vi "Get Last PString.vi"(0 "String":string) -> (1 "Last PString":string, 2 "PString Offset":i32)   [LabVIEW 2017, in "_reuse_openG.lvlib"]
doc: "Returns the last PString from the end of the string and the offset of the beginning of the string."
uses:
  _reuse_openG.lvlib
panel:
  # "[OpenG VI Tags] ***Do Not Remove***"
  # "Get Last PString.vi\n\nReturns the last PString from the end of the string and the offset of the beginn\n\nPlease visit http://www.OpenG.org to learn about the\nOpen Source LabVIEW software movement.\n\nNOTICE -- YOU MUST LEAVE THIS NOTICE IN PLACE.  PER THE TERMS OF THE LICENSE BELOW, YOU MAY SUBLICENSE THIS SOFTWARE \nIN ANY WAY THAT DOES NOT CONFLICT WITH THIS LICENSE.\n\n### BSD License (http://www.opensource.org/licenses/bsd-license.php) Begin ###\n \nCopyright (c) 2002, Jean-Pierre Drolet <drolet_jp@hotmail.com>\nCopyright (c) 2002-2006, Jim Kring <jim@jimkring.com>\n\nAll rights reserved.\n\nRedistribution and use in source and binary forms, with or without modification, are permitted provided that the following conditions are met:\n\n    * Redistributions of source code must retain the above copyright notice, this list of conditions and the following disclaimer.\n    * Redistributions in binary form must reproduce the above copyright notice, this list of conditions and the following disclaimer in the \n       documentation and/or other materials provided with the distribution.\n    * Neither the name of SciWare, James Kring, Inc., nor the names of its contributors may be used to endorse or promote products derived \n       from this software without specific prior written permission.\n\nTHIS SOFTWARE IS PROVIDED BY THE COPYRIGHT HOLDERS AND CONTRIBUTORS \"AS IS\" AND ANY EXPRESS OR IMPLIED WARRANTIES, \nINCLUDING, BUT NOT LIMITED TO, THE IMPLIED WARRANTIES OF MERCHANTABILITY AND FITNESS FOR A PARTICULAR PURPOSE ARE \nDISCLAIMED. IN NO EVENT SHALL THE COPYRIGHT OWNER OR CONTRIBUTORS BE LIABLE FOR ANY DIRECT, INDIRECT, INCIDENTAL,\n SPECIAL, EXEMPLARY, OR CONSEQUENTIAL DAMAGES (INCLUDING, BUT NOT LIMITED TO, PROCUREMENT OF SUBSTITUTE GOODS OR \nSERVICES; LOSS OF USE, DATA, OR PROFITS; OR BUSINESS INTERRUPTION) HOWEVER CAUSED AND ON ANY THEORY OF LIABILITY, \nWHETHER IN CONTRACT, STRICT LIABILITY, OR TORT (INCLUDING NEGLIGENCE OR OTHERWISE) ARISING IN ANY WAY OUT OF THE USE \nOF THIS SOFTWARE, EVEN IF ADVISED OF THE POSSIBILITY OF SUCH DAMAGE.\n\n### BSD License End ###"
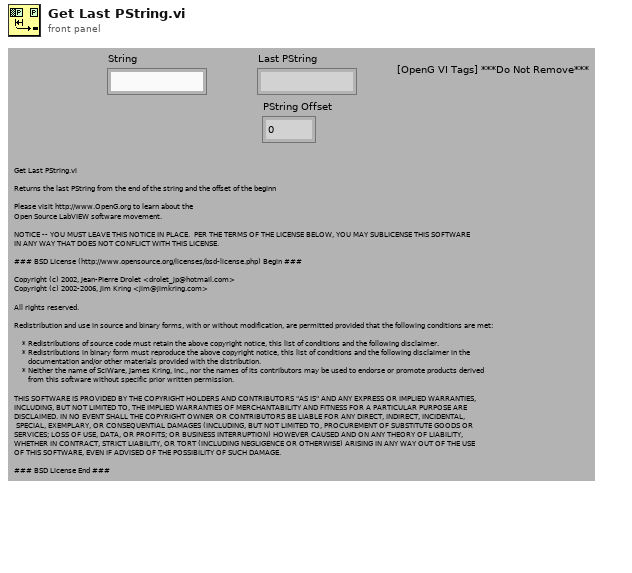
[diagram p1: front panel]
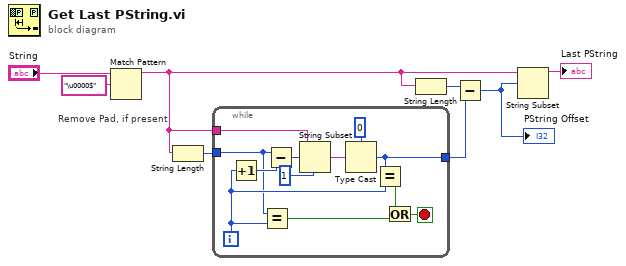
[diagram p0: block diagram]
diagram:
  # "Remove Pad, if present"
  n1 = Match Pattern(string="String", regular expression="\u0000$" ("*(type *) &x")) -> (before substring=w6:string)  [unwired: 1 in, 3 out]
  n2 = String Length(string=w6) -> (length=w7:i32)
  n3 = while {
    tunnel: [w15] -> w1
    tunnel: w7 -> [w10]
    tunnel: w6 -> [w19]
    i -> [w13]
    stop <- w12 stop-if-true
    n4 = Increment(x=w13) -> (x+1=w14:i32)
    n5 = Equal?(x=w10, y=w13) -> (x = y?=w9:bool)
    n6 = Subtract(x=w10, y=w14) -> (x-y=w18:i32)
    n7 = String Subset(string=w19, offset (0)=w18, length (rest)=1 ("length (rest)")) -> (substring=w17:string)
    n8 = Type Cast(type=u8 0, x=w17) -> (*(type *) &x=w15:u8)
    n9 = Equal?(x=w15, y=w13) -> (x = y?=w11:bool)
    n10 = Or(x=w11, y=w9) -> (x .or. y?=w12:bool)
  }
  n11 = String Length(string=w6) -> (length=w4:i32)
  n12 = Subtract(x=w4, y=w1) -> (x-y=w2:i32)
  "PString Offset" <- w2
  n13 = String Subset(string=w6, offset (0)=w2) -> (substring=→"Last PString":string)  [unwired: 1 in]
